vi "Format Body.vi"(4 "Indent":string, 6 "Name":string, 7 "Meta Data":string, 8 "Header":string, 9 "Attributes":string, 10 "Body":string, 11 "IPersist in":refnum<class "IPersist.lvclass">) -> (1 "String out":string, 3 "IPersist out":refnum<class "IPersist.lvclass">)   [LabVIEW 2020, in "IPersist.lvlib" / "IPersist.lvclass"]
uses:
  <vilib>/gpm_packages/@cs/persistence/source/IPersist/IPersist.lvclass
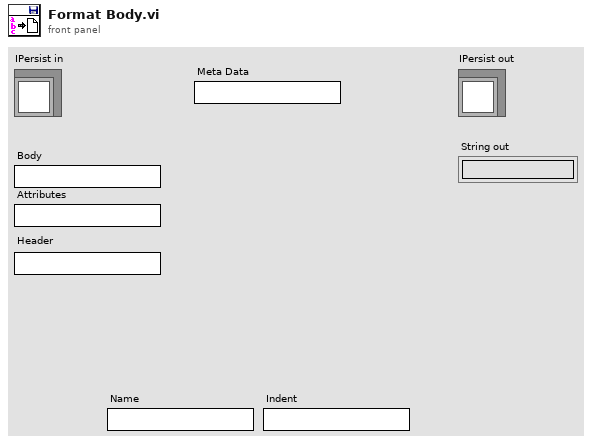
[diagram p1: front panel]
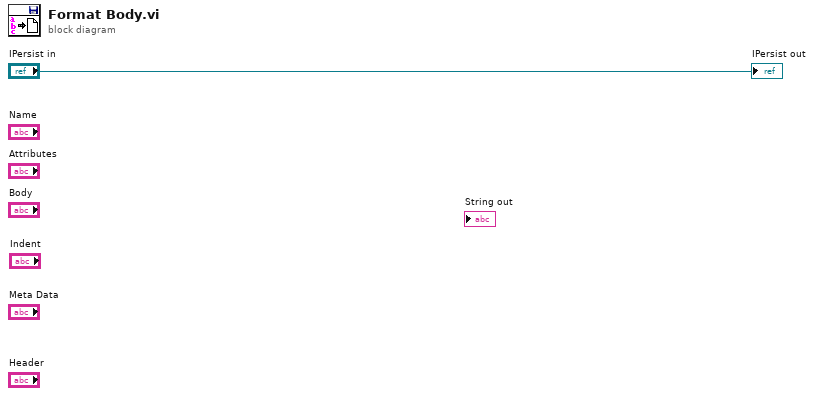
[diagram p0: block diagram]
diagram:
  "IPersist out" <- "IPersist in"
